vi "beta.vi"(1 "alpha":dbl=10.0 format="%#_16g", 2 "NuOptRe":dbl format="%#_16g", 3 "GammaD":dbl format="%#_16g") -> (0 "nuR":dbl format="%#_16g")   [LabVIEW 2015]
panel:
  # "Beta-Correction Function"
  # "Subroutine to compute beta-correction used for hard-collision based line-shape profiles to correct NuOptRe value in the profile. Applicable up to alpha = 5.0, for higher alpha values correction neglected. \nSource: 10.1016/j.jqsrt.2019.106784\n\nStandard Input Parameters:\n--------------------\nGammaD  : Doppler broadening in cm-1. \nNuOptRe : Real part of the Dicke parameter in cm-1.\nalpha   : Mass ratio in the molecule, applicable up to alpha=5, dimensionless.\n\nThe function has one output:\n--------------------\n(1)       : Value of the beta correction, dimensionless."
  # "Input Section"
  # "Output Section"
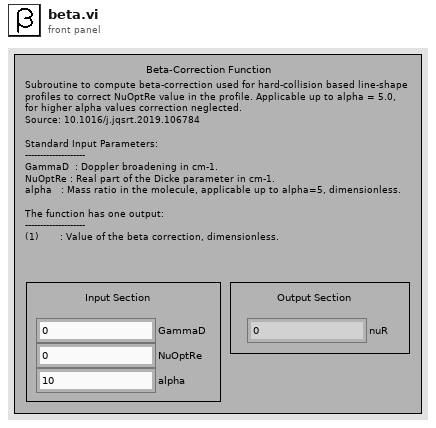
[diagram p1: front panel]
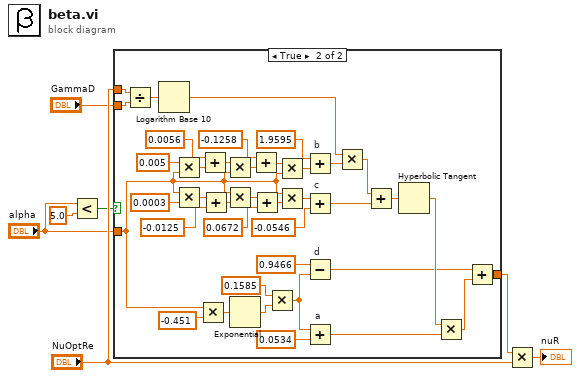
[diagram p0: block diagram]
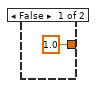
[diagram p2: hidden frame]
diagram:
  n1 = Less?(x="alpha", y=5.0) -> (x < y?=w1:bool)
  n2 = case shown="True" w1 {
    tunnel: [1.0 w9] -> w2
    tunnel: "alpha" -> [_ w31]
    tunnel: "NuOptRe" -> [_ w21]
    tunnel: "GammaD" -> [_ w20]
    frame False {
    }
    frame True {
      n3 = Divide(x=w21, y=w20) -> (x/y=w19:dbl)
      n4 = Logarithm Base 10(1:w19) -> (0:w17:dbl)
      n5 = Multiply(x=0.005, y=w31) -> (x*y=w39:dbl)
      n6 = Multiply(x=w31, y=0.0003) -> (x*y=w29:dbl)
      n7 = Multiply(x=w31, y=-0.451) -> (x*y=w46:dbl)
      n8 = Add(x=0.0056, y=w39) -> (x+y=w37:dbl)
      n9 = Add(x=w29, y=-0.0125) -> (x+y=w28:dbl)
      n10 = Multiply(x=w37, y=w31) -> (x*y=w36:dbl)
      n11 = Multiply(x=w31, y=w28) -> (x*y=w27:dbl)
      n12 = Exponential(1:w46) -> (0:w44:dbl)
      n13 = Add(x=-0.1258, y=w36) -> (x+y=w34:dbl)
      n14 = Add(x=w27, y=0.0672) -> (x+y=w26:dbl)
      n15 = Multiply(x=0.1585, y=w44) -> (x*y=w42:dbl)
      n16 = Multiply(x=w34, y=w31) -> (x*y=w33:dbl)
      n17 = Multiply(x=w31, y=w26) -> (x*y=w25:dbl)
      n18 = Add "b"(x=1.9595, y=w33) -> (x+y=w18:dbl)
      n19 = Add "c"(x=w25, y=-0.0546) -> (x+y=w15:dbl)
      n20 = Subtract "d"(x=0.9466, y=w42) -> (x-y=w11:dbl)
      n21 = Add "a"(x=w42, y=0.0534) -> (x+y=w13:dbl)
      n22 = Multiply(x=w17, y=w18) -> (x*y=w16:dbl)
      n23 = Add(x=w16, y=w15) -> (x+y=w14:dbl)
      n24 = Hyperbolic Tangent(1:w14) -> (0:w12:dbl)
      n25 = Multiply(x=w12, y=w13) -> (x*y=w10:dbl)
      n26 = Add(x=w11, y=w10) -> (x+y=w9:dbl)
    }
  }
  n27 = Multiply(x=w2, y="NuOptRe") -> (x*y=→"nuR":dbl)
